vi "Weather Station UI.vi"(7 "stop":bool, 9 "Limite inférieure":dbl=10.0 min=0.0 max=50.0, 10 "Limite supérieure":dbl=30.0 min=0.0 max=50.0) -> (1 "Mise en garde":string, 2 "Historique de la température":dbl(graph))   [LabVIEW 2009]
doc: "Ceci est le VI principal du Projet Station météo. Il comporte l'interface utilisateur d'un système de mise en garde concernant la température. La température est mesurée toutes les demi-secondes ; les données sont enregistrées lorsqu'une mise en garde survient.\n\nEntrées utilisateur : Limite supérieure de température, Limite inférieure de température, Unités de température.\nSorties : Température actuelle, État de mise en garde."
uses:
  Supporting Files/Weather Station States.ctl
  Instance           1 26Saved   Weather Station UI .vi
panel:
  # "Gamme de température (C)"
  # "Canicule"
  # "Gel"
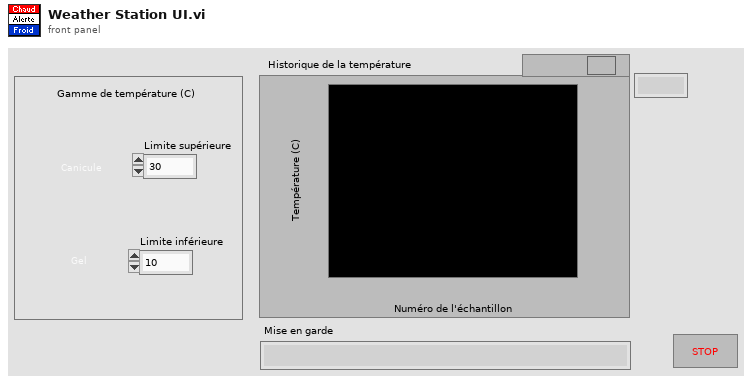
[diagram p1: front panel]
types:
  T1 = enum16{"open", "replace", "create", "open or create", "replace or create", "replace or create with confirmation"}
  T2 = typedef "Weather Station States.ctl" = enum16{"Acquisition", "Analyse", "Enregistrement des données", "Vérification du temps écoulé"}
  T3 = cluster{"Température":dbl, "Limite supérieure de T":dbl, "Limite inférieure de T":dbl, "Mise en garde":string}
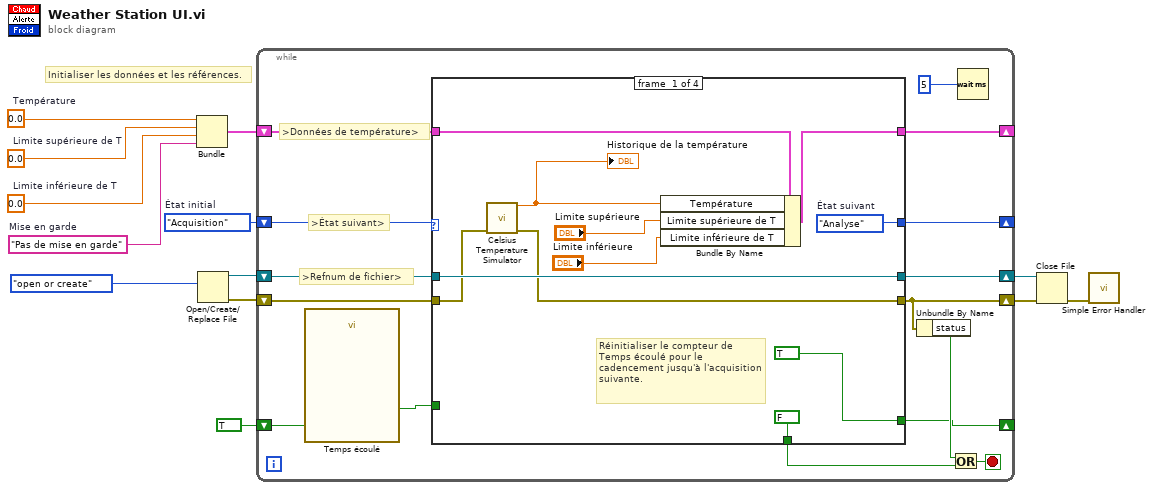
[diagram p0: block diagram]
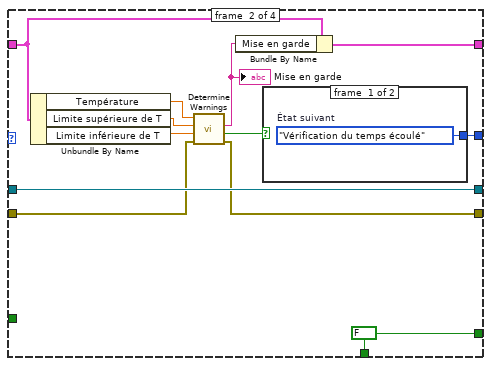
[diagram p2: hidden frame]
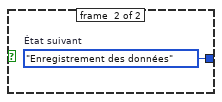
[diagram p3: hidden frame]
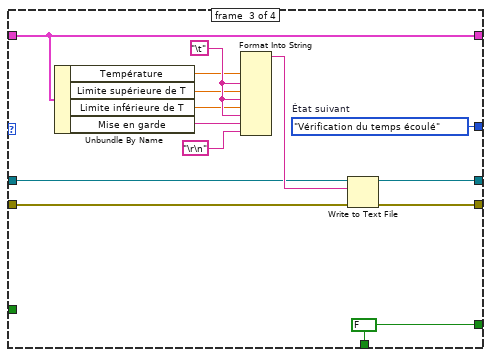
[diagram p4: hidden frame]
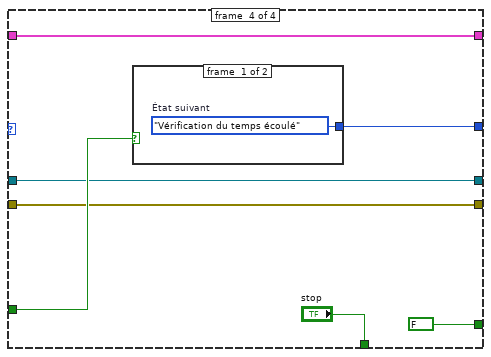
[diagram p5: hidden frame]
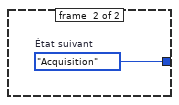
[diagram p6: hidden frame]
diagram:
  w7 = 0.0  # Limite inférieure de T
  w6 = 0.0  # Limite supérieure de T
  w8 = "Pas de mise en garde"  # Mise en garde
  w4 = 0.0  # Température
  w13 = Weather_Station_States."Acquisition"  # État initial
  # "Initialiser les données et les références."
  n1 = Bundle ("Assembler")("Température"=w4, "Limite supérieure de T"=w6, "Limite inférieure de T"=w7, "Mise en garde"=w8) -> (w1:T3)  [unwired: 1 out]
  n2 = Open/Create/Replace File ("Ouvrir/Créer/Remplacer un fichier")(operation (0:open)=T1."open or create") -> (refnum out=w3:refnum<file>, error out=w2:errorcluster)  [unwired: 1 in, 5 out]
  n3 = while "Boucle While" {
    shift-right: [w27] -> _
    shift-left: w13 -> [w28]
    shift-right: [w24] -> w12
    shift-left: w2 -> [w26]
    shift-right: [w14] -> _
    shift-left: w1 -> [w21]
    shift-right: [w22] -> w11
    shift-left: w3 -> [w20]
    shift-right: [w15] -> _
    shift-left: TRUE ("stop") -> [w17]
    stop <- w25 stop-if-true
    # ">Données de température>"
    # ">Refnum de fichier>"
    # ">État suivant>"
    n4 = call "Temps écoulé"("Reset"=w17) -> ("Time has Elapsed"=w16:bool)  [unwired: 4 in, 14 out]
    n5 = case "Structure Condition" shown="\"Acquisition\"" w28 {
      tunnel: [w39 w49 w67 w73] -> w27
      tunnel: [w29 w42 w65 w69] -> w24
      tunnel: w26 -> [w30 w43 w66 w69]
      tunnel: [w38 w51 w64 w70] -> w22
      tunnel: [w32 w44 w54 w68] -> w14
      tunnel: w21 -> [w35 w45 w54 w68]
      tunnel: w20 -> [w38 w51 w62 w70]
      tunnel: [FALSE ("stop") w50 w60 "stop"] -> w19
      tunnel: w16 -> [_ _ _ w74]
      tunnel: [TRUE ("stop") w50 w60 FALSE ("stop")] -> w15
      frame #0 {
        w39 = Weather_Station_States."Analyse"  # État suivant
        # "Réinitialiser le compteur de Temps écoulé pour le cadencement jusqu'à l'acquisition suivante."
        n6 = call "Celsius Temperature Simulator.vi"("entrée d'erreur (pas d'erreur)"=w30) -> ("Température"=w31:dbl, "sortie d'erreur"=w29:errorcluster)  [unwired: 13 out]
        "Historique de la température" <- w31
        n7 = Bundle By Name(cluster=w35, "Température"=w31, "Limite supérieure de T"="Limite supérieure", "Limite inférieure de T"="Limite inférieure") -> (w32:T3)
      }
      frame #1 {
        w50 = FALSE ("stop")
        n8 = Unbundle By Name(w45) -> ("Température"=w48:dbl, "Limite supérieure de T"=w47:dbl, "Limite inférieure de T"=w46:dbl)
        n9 = call "Determine Warnings.vi"("entrée d'erreur (pas d'erreur)"=w43, "Temp. min."=w46, "Temp. max."=w47, "Temp. actuelle"=w48) -> ("sortie d'erreur"=w42:errorcluster, "Mise en garde ?"=w40:bool, "Texte de mise en garde"=w41:string)  [unwired: 5 out]
        "Mise en garde" <- w41
        n10 = Bundle By Name(cluster=w45, "Mise en garde"=w41) -> (w44:T3)
        n11 = case shown="Faux" w40 {
          tunnel: [w52 w53] -> w49
          frame #0 {
            w52 = Weather_Station_States."Vérification du temps écoulé"  # État suivant
          }
          frame #1 {
            w53 = Weather_Station_States."Enregistrement des données"  # État suivant
          }
        }
      }
      frame #2 {
        w67 = Weather_Station_States."Vérification du temps écoulé"  # État suivant
        w60 = FALSE ("stop")
        w61 = "\t"
        n12 = Unbundle By Name(w54) -> ("Température"=w59:dbl, "Limite supérieure de T"=w58:dbl, "Limite inférieure de T"=w57:dbl, "Mise en garde"=w56:string)
        n13 = Format Into String(w59, w61, w58, w61, w57, w61, w56, "\r\n") -> (resulting string=w63:string)  [unwired: 3 in, 1 out]
        n14 = Write to Text File(file (use dialog)=w62, text=w63, error in=w66) -> (refnum out=w64:refnum<file>, error out=w65:errorcluster)  [unwired: 2 out]
      }
      frame #3 {
        n15 = case shown="Faux" w74 {
          tunnel: [w75 w76] -> w73
          frame #0 {
            w75 = Weather_Station_States."Vérification du temps écoulé"  # État suivant
          }
          frame #1 {
            w76 = Weather_Station_States."Acquisition"  # État suivant
          }
        }
      }
    }
    n16 = Unbundle By Name ("Désassembler par nom")(w24) -> ("status"=w23:bool)
    n17 = Or ("OU")(x=w23, y=w19) -> (x .or. y?=w25:bool)
    n18 = Wait (ms) ("Attendre (ms)")(milliseconds to wait=u32 5 ("y")) -> ()  [unwired: 1 out]
  }
  n19 = Close File ("Fermer un fichier")(refnum=w11, error in=w12) -> (error out=w10:errorcluster)  [unwired: 1 out]
  n20 = call <vilib>:"Simple Error Handler.vi"("error in (no error)"=w10) -> ()  [unwired: 1 in, 8 out]
